vi "Build.vi"(6 "Assembly Type":string, 8 "Position":i32, 9 "XYZTheta":dbl[](array[numeric]), 10 "Pattern Coordinates":dbl[][](array[numeric]), 11 "C4 Dispense in":refnum<class "Iterative Dispense.lvclass">) -> (3 "C4 Dispense out":refnum<class "Iterative Dispense.lvclass">)   [LabVIEW 2021, in "Iterative Dispense.lvclass"]
uses:
  Iterative Dispense.lvclass
  C:/Users/HEP/Documents/GitHub/Gantry/UCSB-Gantry-HEP-main/Classes/Routine/Dispense/Dispense.lvclass
  Iterative Dispense.lvclass/Iterative Dispense.ctl
  <vilib>/Analysis/coordinate.llb/2D Cartesian Coordinate Rotation (Array).vi
  <vilib>/Analysis/NI_AALPro.lvlib
panel:
  out "Array":dbl[][][](array[numeric])
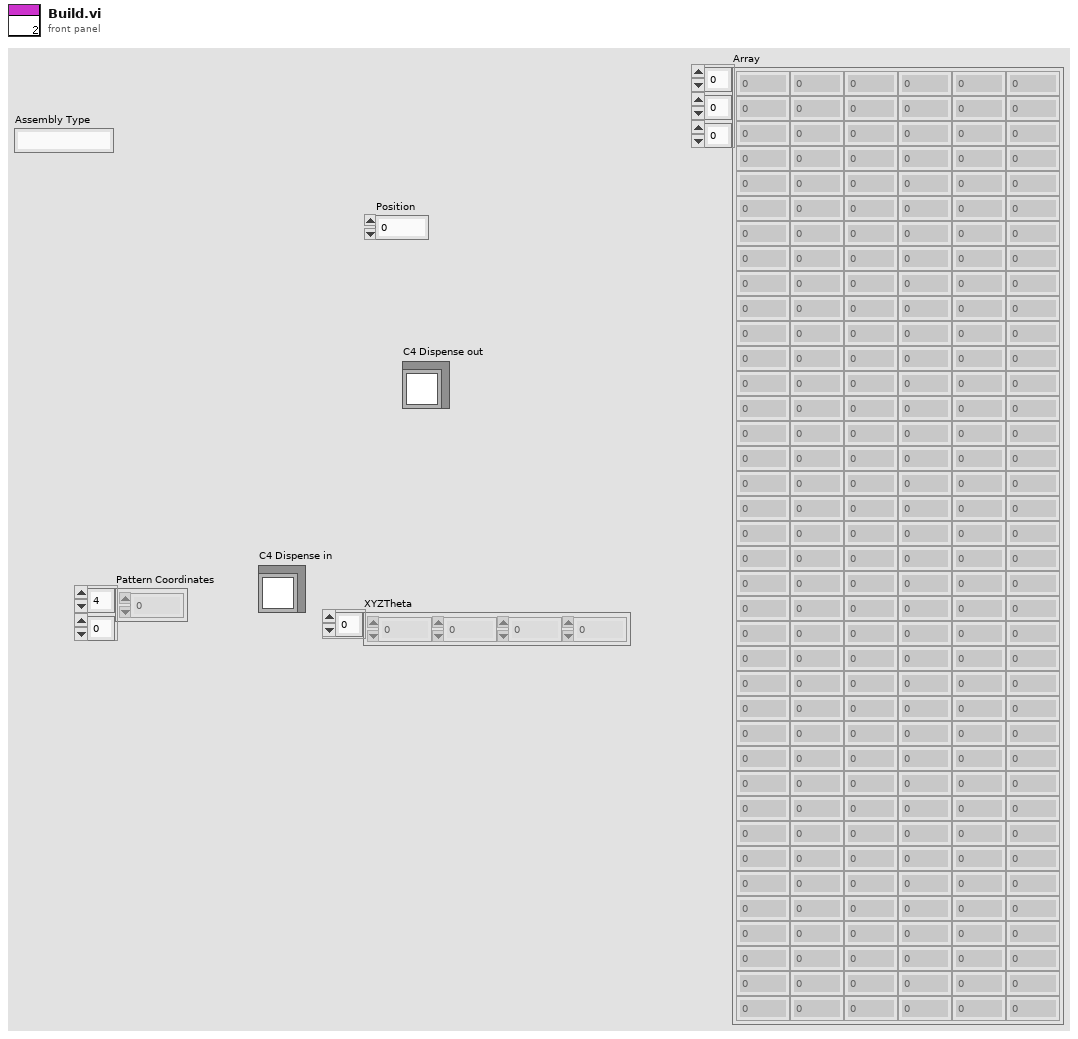
[diagram p1: front panel]
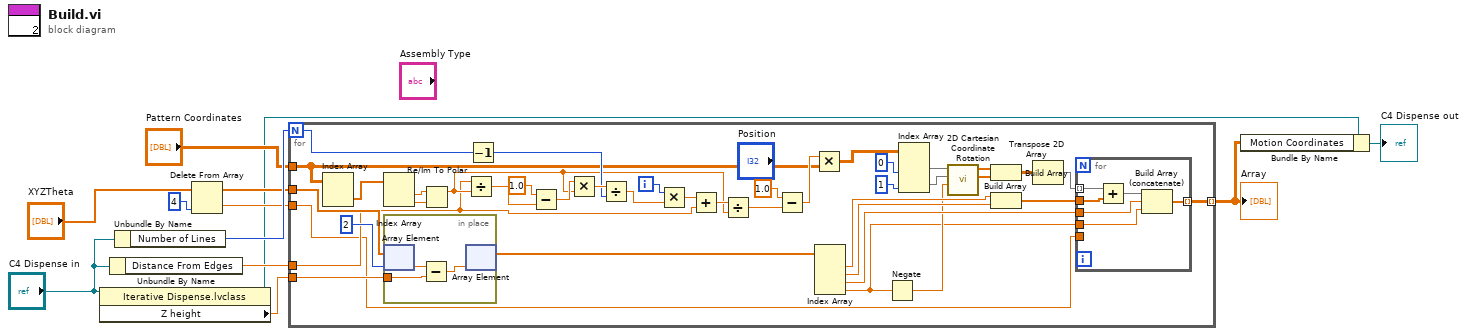
[diagram p0: block diagram]
diagram:
  n1 = property class="Iterative Dispense.lvclass"(reference="C4 Dispense in") -> (reference out=w2:refnum<class "Iterative Dispense.lvclass">, "Z height"=w11:dbl)  [unwired: 1 in, 1 out]
  n2 = Unbundle By Name("C4 Dispense in") -> ("Distance From Edges"=w10:dbl)
  n3 = Unbundle By Name("C4 Dispense in") -> ("Number of Lines"=w12:i32)
  n4 = Delete From Array(array="XYZTheta", index=4) -> (deleted portion=w3:dbl, array with subset deleted=w5:dbl[])  [unwired: 1 in]
  n5 = for {
    N: w12 -> [w33]
    tunnel: w5 -> [w25]
    tunnel: "Pattern Coordinates" -> [w32]
    tunnel: w11 -> [w24]
    tunnel: [w21] -> w8 mode=indexing
    tunnel: w10 -> [w20]
    tunnel: w3 -> [w19]
    i -> [w47]
    n6 = Index Array(array=w32) -> (element=w31:dbl[])  [unwired: 2 in]
    n7 = Index Array(array=w31) -> (element #1=w30:dbl, element #2=w29:dbl)  [unwired: 2 in]
    n8 = in-place {
      in-place-border: w24 -> [w54]
      n9 = in-place-array #1(w25, 2) -> (w55:dbl)
      n10 = Subtract(x=w55, y=w54) -> (x-y=w53:dbl)
      n11 = in-place-array #1(w53) -> (w23:dbl[])  [unwired: 1 out]
    }
    n12 = Re/Im To Polar(2:w29, 3:w30) -> (1:w37:dbl)  [unwired: 1 out]
    n13 = Divide(x=w20, y=w37) -> (x/y=w43:dbl)
    n14 = Decrement(x=w33) -> (x-1=w39:i32)
    n15 = Subtract(x=1.0, y=w43) -> (x-y=w41:dbl)
    n16 = Multiply(x=w41, y=w37) -> (x*y=w40:dbl)
    n17 = Divide(x=w40, y=w39) -> (x/y=w38:dbl)
    n18 = Multiply(x=w47, y=w38) -> (x*y=w52:dbl)
    n19 = Add(x=w52, y=w20) -> (x+y=w51:dbl)
    n20 = Divide(x=w51, y=w37) -> (x/y=w50:dbl)
    n21 = Subtract(x=1.0, y=w50) -> (x-y=w44:dbl)
    n22 = Multiply(x=w44, y=w32) -> (x*y=w48:dbl[][])
    n23 = Index Array(array=w23) -> (element #1=w36:dbl, element #2=w35:dbl, element #3=w22:dbl, element #4=w13:dbl)  [unwired: 4 in]
    n24 = Negate(x=w13) -> (-x=w16:dbl)
    n25 = Index Array(array=w48, index (col) #1=0 ("disabled index (col)"), index (col) #2=1 ("index (col)")) -> (element #1=w18:dbl[], element #2=w17:dbl[])  [unwired: 2 in]
    n26 = call-poly <vilib>:"2D Cartesian Coordinate Rotation.vi"("theta"=w16, "Y"=w17, "X"=w18) -> ("Y Out"=w14:dbl[], "X Out"=w15:dbl[])  [unwired: 6 in, 1 out]
    n27 = Build Array(w15, w14) -> (w28:dbl[][])
    n28 = Build Array(w36, w35) -> (w34:dbl[])
    n29 = Transpose 2D Array(2D array=w28) -> (transposed array=w27:dbl[][])
    n30 = for {
      tunnel: w34 -> [w61]
      tunnel: w27 -> [w60] mode=indexing
      tunnel: w22 -> [w59]
      tunnel: [w58] -> w21 mode=indexing
      tunnel: w19 -> [_]
      tunnel: w13 -> [w56]
      n31 = Add(x=w60, y=w61) -> (x+y=w57:dbl[])
      n32 = Build Array (concatenate)(w57, w59, w56) -> (w58:dbl[])
    }
  }
  "Array" <- w8
  n33 = Bundle By Name(cluster=w2, "Motion Coordinates"=w8) -> (→"C4 Dispense out":refnum<class "Iterative Dispense.lvclass">)
